vi "Lookup Function by Name.vi"(8 "error in (no error)":errorcluster, 10 "Function Name":string, 11 "Controller in":refnum<class "Controller.lvclass">) -> (0 "error out":errorcluster, 1 "found":bool, 2 "Function.lvclass":refnum<class "Function.lvclass">, 3 "Controller out":refnum<class "Controller.lvclass">)   [LabVIEW 2016, in "Controller Actor.lvlib" / "Controller.lvclass"]
uses:
  <userlib>/Common Components/Controller/Controller.lvclass
  <userlib>/Common Components/Function Actor/Function.lvclass
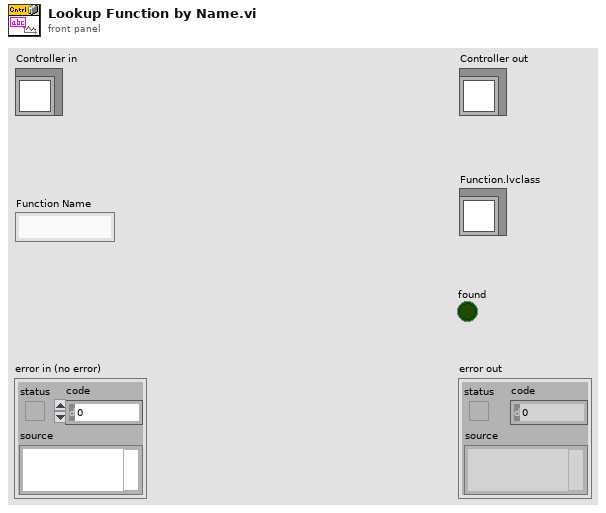
[diagram p1: front panel]
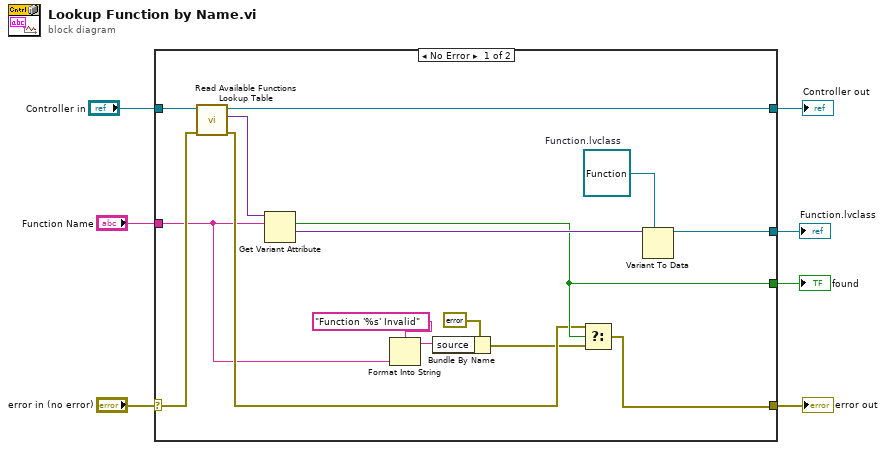
[diagram p0: block diagram]
diagram:
  n1 = case shown="No Error" "error in (no error)" {
    selector: "error in (no error)" -> [w16 w24]
    tunnel: [w9 w24] -> w6
    tunnel: [w20 w23] -> w4
    tunnel: "Controller in" -> [w22 w23]
    tunnel: "Function Name" -> [w8 _]
    tunnel: [w17 _] -> w2
    tunnel: [w12 _] -> w1
    frame No Error {
      w18 = refnum<class "Function.lvclass"> refnum  # Function.lvclass
      n2 = call <userlib>:"Read Available Functions Lookup Table.vi"("error in (no error)"=w16, "Controller in"=w22) -> ("error out"=w11:errorcluster, "Available Functions Lookup Table"=w21:variant, "Controller out"=w20:refnum<class "Controller.lvclass">)  [unwired: 7 in]
      n3 = Get Variant Attribute(Variant=w21, name=w8) -> (found=w12:bool, value=w19:variant)  [unwired: 2 in, 2 out]
      n4 = Format Into String(format string="Function '%s' Invalid" ("source"), w8) -> (resulting string=w14:string)  [unwired: 2 in, 1 out]
      n5 = Bundle By Name(cluster=errorcluster {"status"=TRUE, "code"=5559, "source"="Function '%s' Invalid"} ("error constant"), "source"=w14) -> (w10:errorcluster)
      n6 = Select(t=w11, s=w12, f=w10) -> (s? t:f=w9:errorcluster)
      n7 = Variant To Data(type=w18, Variant=w19) -> (data=w17:refnum<class "Function.lvclass">)  [unwired: 1 in, 1 out]
    }
    frame Error {
    }
  }
  "error out" <- w6
  "Controller out" <- w4
  "Function.lvclass" <- w2
  "found" <- w1
